vi "Find Intersections of Fitted Line with Universal Circle.vi"(8 "Error In":errorcluster, 11 "Phasor Array":T1[](array[typedef])) -> (0 "Error Out":errorcluster, 2 "Point 2":cluster{"x":dbl, "y":dbl}, 3 "Point 1":cluster{"x":dbl, "y":dbl})   [LabVIEW 2019]
uses:
  Phasor (g, s).ctl
  <vilib>/Utility/error.llb/DialogType.ctl
  <vilib>/Analysis/6fits.llb/Curve Fitting Criteria.ctl
  <vilib>/Analysis/NI_AALPro.lvlib
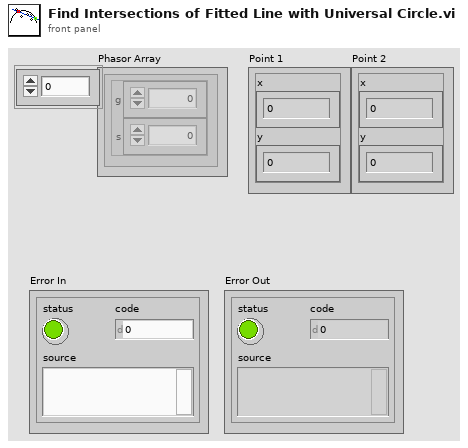
[diagram p1: front panel]
types:
  T1 = typedef "Phasor (g, s).ctl" = cluster{"g":dbl, "s":dbl}
  T2 = typedef "DialogType.ctl" = u16
  T3 = typedef "NI_AALPro.lvlib/Curve Fitting Criteria.ctl" = u16
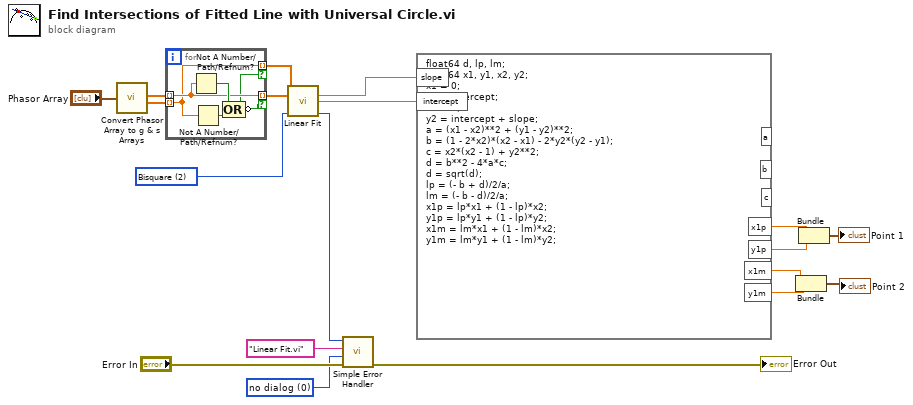
[diagram p0: block diagram]
diagram:
  w5 = T2 0 items=["no dialog", "OK message", "continue or stop message", "OK message + warnings", "continue/stop + warnings"] ("type of dialog (OK msg:1)")
  w11 = T3 2 items=["Least Square", "Least Absolute Residual", "Bisquare"] ("method")
  n1 = call "Convert Phasor Array to g & s Arrays.vi"("Phasor Array"="Phasor Array") -> ("g"=w4:dbl[], "s"=w3:dbl[])  [unwired: 8 in]
  n2 = for {
    tunnel: w4 -> [w22] mode=indexing
    tunnel: w3 -> [w21] mode=indexing
    tunnel: [w22] -> w2 mode=indexing if=w20
    tunnel: [w21] -> w1 mode=indexing if=w20
    n3 = Not A Number/Path/Refnum?(number/path/refnum=w22) -> (NaN/Path/Refnum?=w23:bool)
    n4 = Not A Number/Path/Refnum?(number/path/refnum=w21) -> (NaN/Path/Refnum?=w24:bool)
    n5 = Compound Arithmetic op=OR(w23, w24) -> (invert w20:bool)
  }
  n6 = call <vilib>:"Linear Fit.vi"("Y"=w1, "X"=w2, "method"=w11) -> ("slope"=w10:dbl, "intercept"=w9:dbl, "error"=w7:i32)  [unwired: 8 in, 2 out]
  n7 = call <vilib>:"Simple Error Handler.vi"("error code (no error:0)"=w7, "error source (\" \")"="Linear Fit.vi" ("error source (\" \")"), "type of dialog (OK msg:1)"=w5, "error in (no error)"="Error In") -> ("error out"=→"Error Out":errorcluster)  [unwired: 1 in, 4 out]
  n8 = formula code="float64 d, lp, lm;\nfloat64 x1, y1, x2, y2;\nx1 = 0;\ny1 = intercept;\nx2 = 1;\ny2 = intercept + slope;\na = (x1 - x2)**2 + (y1 - y2)**2;\nb = (1 - 2*x2)*(x2 - x1) - 2*y2*(y2 - y1);\nc = x2*(x2 - 1) + y2**2;\nd = b**2 - 4*a*c;\nd = sqrt(d);\nlp = (- b + d)/2/a;\nlm = (- b - d)/2/a;\nx1p = lp*x1 + (1 - lp)*x2;\ny1p = lp*y1 + (1 - lp)*y2;\nx1m = lm*x1 + (1 - lm)*x2;\ny1m = lm*y1 + (1 - lm)*y2;"("slope"=w10, "intercept"=w9) -> ("x1p"=w19:dbl, "x1m"=w16:dbl, "y1p"=w18:dbl, "y1m"=w15:dbl)  [unwired: 3 out]
  n9 = Bundle("x1m"=w16, "y1m"=w15) -> (→"Point 2":cluster{"x1m":dbl, "y1m":dbl})  [unwired: 1 in]
  n10 = Bundle("x1p"=w19, "y1p"=w18) -> (→"Point 1":cluster{"x1p":dbl, "y1p":dbl})  [unwired: 1 in]
